vi "test_integration_decodage.vi"() -> ()   [LabVIEW 2018]
panel:
  in  "sigma2":string
  out "vec bits décodés":i8[](array[numeric])
  out "sortie décodeur":string
  out "sortie complexe":string
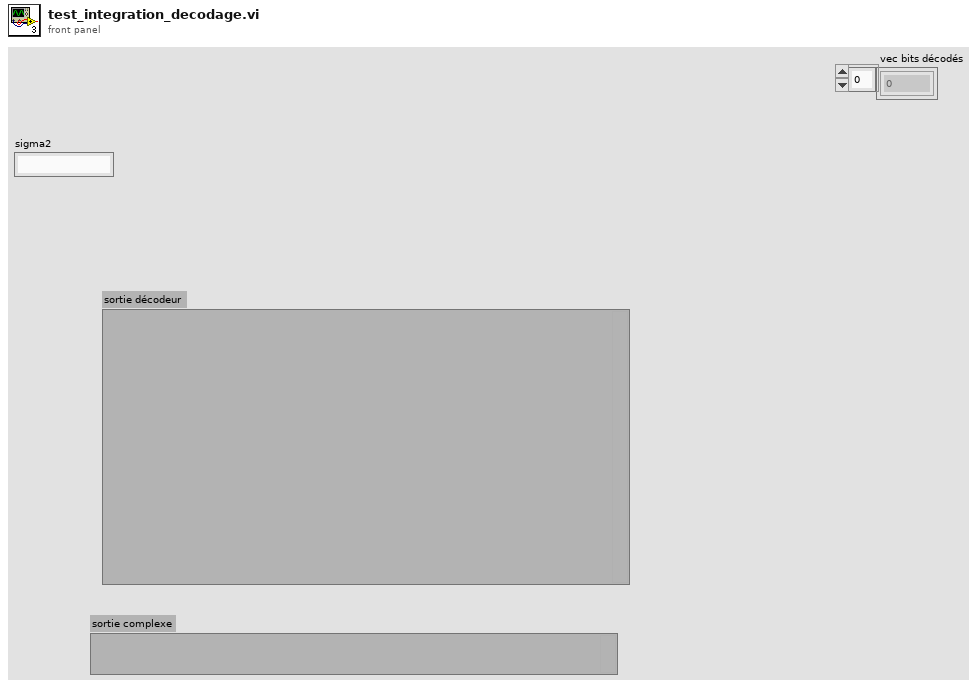
[diagram p1: front panel]
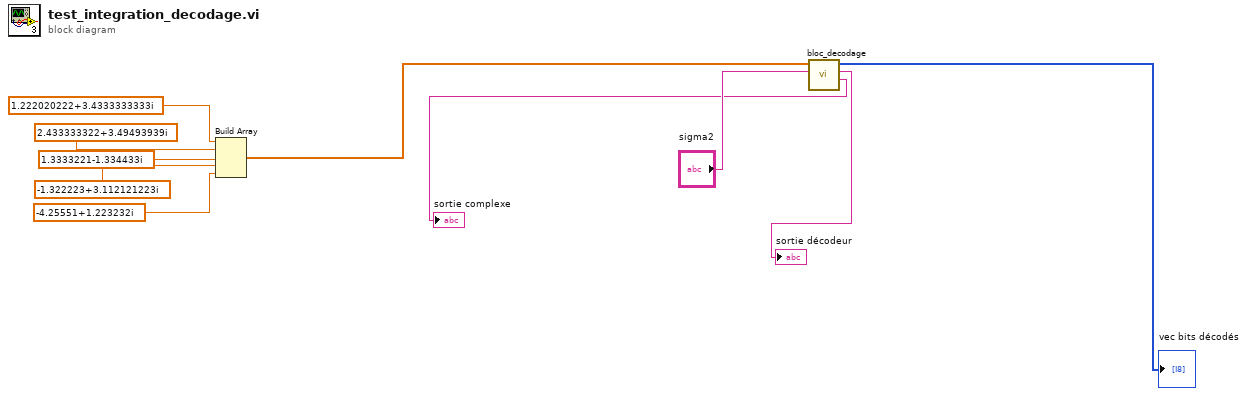
[diagram p0: block diagram]
diagram:
  n1 = Build Array(cdb 1.222020222+3.4333333333i, cdb 2.433333322+3.49493939i, cdb 1.3333221-1.334433i, cdb -1.322223+3.112121223i, cdb -4.25551+1.223232i) -> (w5:cdb[])
  n2 = call "bloc_decodage.vi"("sigma2"="sigma2", "Array"=w5) -> ("sortie complexe"=→"sortie complexe":string, "sortie décodeur"=→"sortie décodeur":string, "output bit stream"=→"vec bits décodés":i8[])  [unwired: 7 in]
